vi "config.vi"() -> ()   [LabVIEW 2016]
panel:
  in  "User Defined Ramp Rate (T/min)":dbl=0.145
  in  "TController Stability (K)":dbl=0.01
  out "Max Ramp Rate Z-Axis (A/s)":dbl=0.19
  out "Max Ramp Rate Y-Axis (A/s)":dbl=0.055
  in  "Z-Axis Communications Config":T1={"GPIB address"=22, "GPIB bus"=0, "connection ID"=refnum, "IP"="111.111.111.1", "Active Comm Interface"=0, "Serial Port"="", "Programmer Type"=0} {"Programmer Type" items=["Model 430", "Model 420"]; "Active Comm Interface" items=["TCP/IP (Model 430 Only)", "RS232", "IEEE488"]}
  in  "Y-Axis Communications Config":T1={"GPIB address"=22, "GPIB bus"=0, "connection ID"=refnum, "IP"="111.111.111.2", "Active Comm Interface"=0, "Serial Port"="", "Programmer Type"=0} {"Programmer Type" items=["Model 430", "Model 420"]; "Active Comm Interface" items=["TCP/IP (Model 430 Only)", "RS232", "IEEE488"]}
  in  "TController Sample Input":u8(ring)=1 items=["ChA", "ChB", "ChC", "ChD"]
  in  "TController Sample Output":u8(ring) items=["Loop 1", "Loop 2"]
  in  "TController Stability Count":i32=3
  in  "TController Stability Delay (ms)":i32=5000
  in  "GPIB VNA":refnum<visa-resource-name>="GPIB1::16::INSTR"
  in  "Magnet Device":enum16{"ips120", "amiVector"}(ring)=enum."amiVector"
  in  "GPIB IPS120 MagnetPSU":refnum<visa-resource-name>="COM1"
  in  "GPIB Cryocon32B":refnum<visa-resource-name>="GPIB1::12::INSTR"
  in  "GPIB Gaussmeter":refnum<visa-resource-name>="GPIB1::11::INSTR"
  # "GPIB Identifiers for Devices"
  # "Select which magnet to use:"
  # "Temperature Controller Settings.\n======================"
  # "Stability interval required to start the measurement."
  # "Time to wait between consecutive T measurements."
  # "Number of measurements which have to fall in a certain\nrange to consider the temperature as stable."
  # "Output loop and input channel of the sample temperature\nsensor/heater."
  # "AMI Magnet\n========="
  # "These are the rates specified by AMI and are \nNOT to be exceeded!!"
  # "0.150 T/min corresponds to 0.055 A/s for the Y-coil. As soon as this rate is exceed, the Z-coil will sweep faster than the Y-coil and the field vector does not rotate uniformly!"
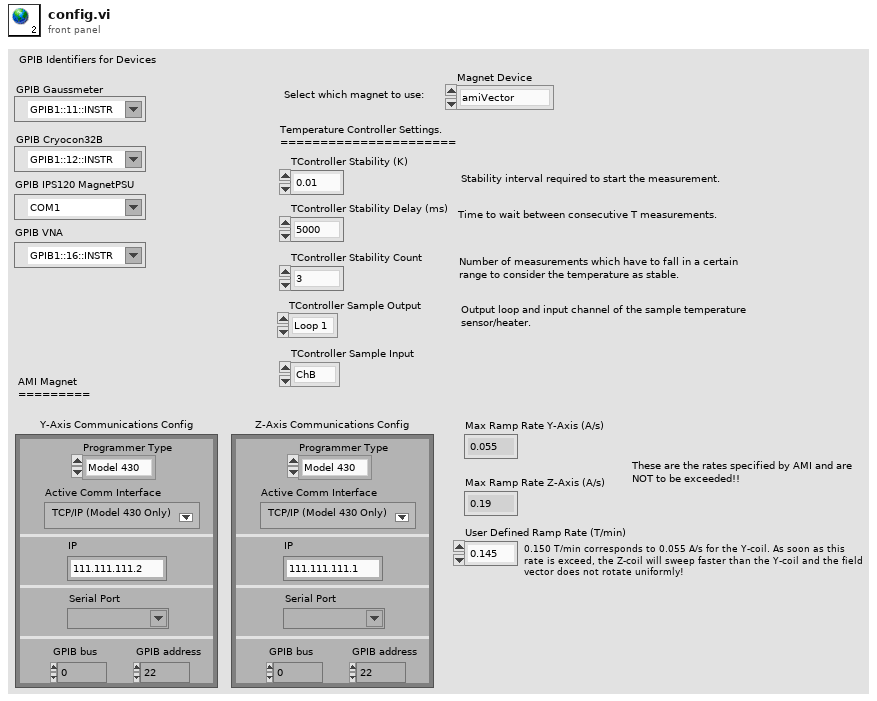
[diagram p1: front panel]
types:
  T1 = cluster{"GPIB address":i16, "GPIB bus":i16, "connection ID":refnum<k5>, "IP":string, "Active Comm Interface":u16, "Serial Port":refnum<visa-resource-name>, "Programmer Type":u16}
diagram:
